vi "StartRecorder.vi"(0 "axis in":cluster{"keyHandle":u32, "nodeId":u16}={"keyHandle"=0, "nodeId"=1}, 5 "parameter":T2, 7 "trigger type":u8(ring)=1 items=["movement start trigger"=1, "error trigger"=2, "digital input trigger"=4, "movement end trigger"=8], 9 "recorded objects":T1 {"recorded object 4"."objectSubIndex" format="%x"; "recorded object 4"."objectIndex" format="%x"; "recorded object 3"."objectSubIndex" format="%x"; "recorded object 3"."objectIndex" format="%x"; "recorded object 2"."objectSubIndex" format="%x"; "recorded object 2"."objectIndex" format="%x"; "recorded object 1"."objectSubIndex" format="%x"; "recorded object 1"."objectIndex" format="%x"}, 11 "error in (no error)":errorcluster) -> (4 "axis out":cluster{"keyHandle":u32, "nodeId":u16}={"keyHandle"=0, "nodeId"=1}, 15 "error out":errorcluster)   [LabVIEW 2018]
doc: "<B>StartRecorder</B> writes the data recorder parameters and the trigger type. The channels 1 - 4 can be activated. After correct parameter configuration the data recorder is started."
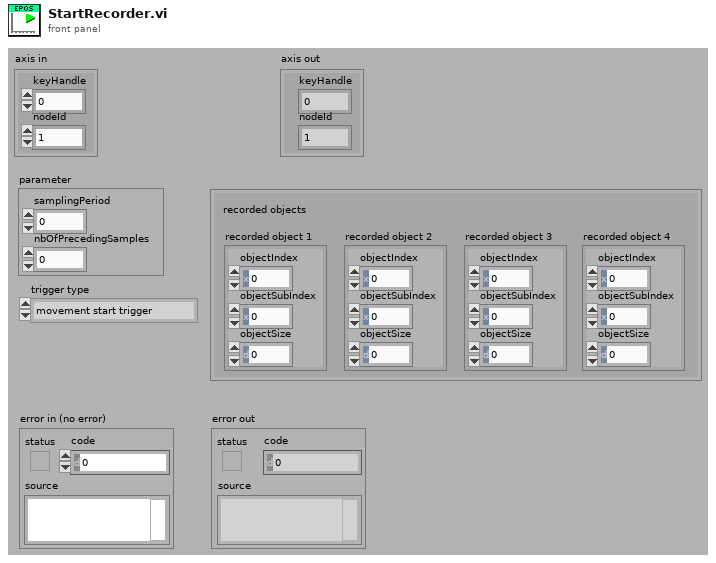
[diagram p1: front panel]
types:
  T1 = cluster{"recorded object 1":cluster{"objectIndex":u16, "objectSubIndex":u8, "objectSize":u8}, "recorded object 2":cluster{"objectIndex":u16, "objectSubIndex":u8, "objectSize":u8}, "recorded object 3":cluster{"objectIndex":u16, "objectSubIndex":u8, "objectSize":u8}, "recorded object 4":cluster{"objectIndex":u16, "objectSubIndex":u8, "objectSize":u8}}
  T2 = cluster{"samplingPeriod":u16, "nbOfPrecedingSamples":u16}
  T3 = cluster{"objectIndex":u16, "objectSubIndex":u8, "objectSize":u8}
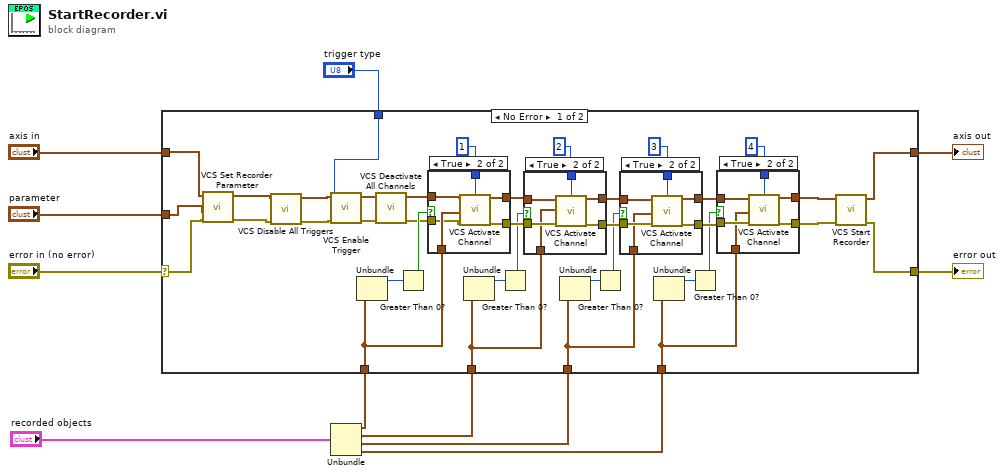
[diagram p0: block diagram]
diagram:
  n1 = Unbundle("recorded objects") -> ("recorded object 1"=w4:T3, "recorded object 2"=w3:T3, "recorded object 3"=w2:T3, "recorded object 4"=w1:T3)
  n2 = case shown="No Error" "error in (no error)" {
    selector: "error in (no error)" -> [w13 w83]
    tunnel: [w33 w83] -> w10
    tunnel: [w31 w82] -> w9
    tunnel: "axis in" -> [w14 w82]
    tunnel: "parameter" -> [w12 _]
    tunnel: "trigger type" -> [w49 _]
    tunnel: w4 -> [w26 _]
    tunnel: w3 -> [w25 _]
    tunnel: w2 -> [w24 _]
    tunnel: w1 -> [w23 _]
    frame No Error {
      n3 = call "VCS Set Recorder Parameter.vi"("error in (no error)"=w13, "parameter"=w12, "axis in"=w14) -> ("error out"=w17:errorcluster, "axis out"=w15:cluster{"keyHandle":u32, "nodeId":u16})  [unwired: 7 in]
      n4 = call "VCS Disable All Triggers.vi"("error in (no error)"=w17, "axis in"=w15) -> ("error out"=w18:errorcluster, "axis out"=w16:cluster{"keyHandle":u32, "nodeId":u16})  [unwired: 8 in]
      n5 = call "VCS Enable Trigger.vi"("error in (no error)"=w18, "trigger type"=w49, "axis in"=w16) -> ("error out"=w21:errorcluster, "axis out"=w22:cluster{"keyHandle":u32, "nodeId":u16})  [unwired: 7 in]
      n6 = Unbundle(w26) -> ("objectIndex"=w30:u16)  [unwired: 2 out]
      n7 = call "VCS Deactivate All Channels.vi"("error in (no error)"=w21, "axis in"=w22) -> ("error out"=w19:errorcluster, "axis out"=w20:cluster{"keyHandle":u32, "nodeId":u16})  [unwired: 8 in]
      n8 = Greater Than 0?(x=w30) -> (x > 0?=w47:bool)
      n9 = case shown="True" w47 {
        tunnel: u8 1 ("channelNumber") -> [_ w81]
        tunnel: [w75 w80] -> w39
        tunnel: [w74 w79] -> w40
        tunnel: w26 -> [_ w78]
        tunnel: w20 -> [w74 w77]
        tunnel: w19 -> [w75 w76]
        frame False {
        }
        frame True {
          n10 = call "VCS Activate Channel.vi"("axis in"=w77, "channelNumber"=w81, "recorded object"=w78, "error in (no error)"=w76) -> ("axis out"=w79:cluster{"keyHandle":u32, "nodeId":u16}, "error out"=w80:errorcluster)  [unwired: 14 in]
        }
      }
      n11 = Unbundle(w25) -> ("objectIndex"=w29:u16)  [unwired: 2 out]
      n12 = Greater Than 0?(x=w29) -> (x > 0?=w37:bool)
      n13 = case shown="True" w37 {
        tunnel: u8 2 ("channelNumber") -> [_ w73]
        tunnel: w39 -> [w66 w72]
        tunnel: [w66 w71] -> w42
        tunnel: w40 -> [w67 w70]
        tunnel: [w67 w69] -> w41
        tunnel: w25 -> [_ w68]
        frame False {
        }
        frame True {
          n14 = call "VCS Activate Channel.vi"("axis in"=w70, "channelNumber"=w73, "recorded object"=w68, "error in (no error)"=w72) -> ("axis out"=w69:cluster{"keyHandle":u32, "nodeId":u16}, "error out"=w71:errorcluster)  [unwired: 14 in]
        }
      }
      n15 = Unbundle(w24) -> ("objectIndex"=w28:u16)  [unwired: 2 out]
      n16 = Greater Than 0?(x=w28) -> (x > 0?=w36:bool)
      n17 = case shown="True" w36 {
        tunnel: u8 3 ("channelNumber") -> [_ w65]
        tunnel: w42 -> [w58 w64]
        tunnel: [w58 w63] -> w38
        tunnel: w41 -> [w59 w62]
        tunnel: [w59 w61] -> w43
        tunnel: w24 -> [_ w60]
        frame False {
        }
        frame True {
          n18 = call "VCS Activate Channel.vi"("axis in"=w62, "channelNumber"=w65, "recorded object"=w60, "error in (no error)"=w64) -> ("axis out"=w61:cluster{"keyHandle":u32, "nodeId":u16}, "error out"=w63:errorcluster)  [unwired: 14 in]
        }
      }
      n19 = Unbundle(w23) -> ("objectIndex"=w27:u16)  [unwired: 2 out]
      n20 = Greater Than 0?(x=w27) -> (x > 0?=w35:bool)
      n21 = case shown="True" w35 {
        tunnel: u8 4 ("channelNumber") -> [_ w57]
        tunnel: w38 -> [w50 w56]
        tunnel: [w50 w55] -> w34
        tunnel: w43 -> [w51 w54]
        tunnel: [w51 w53] -> w32
        tunnel: w23 -> [_ w52]
        frame False {
        }
        frame True {
          n22 = call "VCS Activate Channel.vi"("axis in"=w54, "channelNumber"=w57, "recorded object"=w52, "error in (no error)"=w56) -> ("axis out"=w53:cluster{"keyHandle":u32, "nodeId":u16}, "error out"=w55:errorcluster)  [unwired: 14 in]
        }
      }
      n23 = call "VCS Start Recorder.vi"("error in (no error)"=w34, "axis in"=w32) -> ("error out"=w33:errorcluster, "axis out"=w31:cluster{"keyHandle":u32, "nodeId":u16})  [unwired: 8 in]
    }
    frame Error {
    }
  }
  "error out" <- w10
  "axis out" <- w9
